vi "Configure Power Meter Settings.vi"(0 "VISA resource name":refnum<visa-resource-name>, 1 "Power Meter Average Count (10)":i32=10 min=2 max=1000, 2 "Power Meter Average State (0:Off)":i32(ring) items=["Off", "On"], 5 "Power Meter Frequency (1000000000Hz)":dbl=1000000000.0, 7 "Power Meter Offset State (0:Off)":i32(ring) items=["Off", "On"], 9 "Power Meter Offset (0.00dB)":dbl min=-100.0 max=100.0 step=0.01 format="%.2f", 11 "error in (no error)":errorcluster, 12 "Power Meter Range (0:Auto)":i32(ring) items=["Auto", "Low", "High"]) -> (4 "VISA resource name out":refnum<visa-resource-name>, 15 "error out":errorcluster)   [LabVIEW 2020, in "Anritsu Signal Analyzer Series.lvlib"]
doc: "Configures the Power Meter settings."
uses:
  Anritsu Signal Analyzer Series.lvlib
panel:
  # "Hz"
  # "dB"
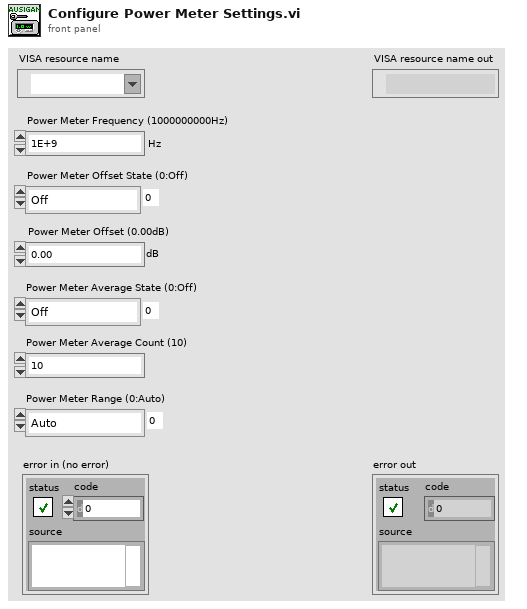
[diagram p1: front panel]
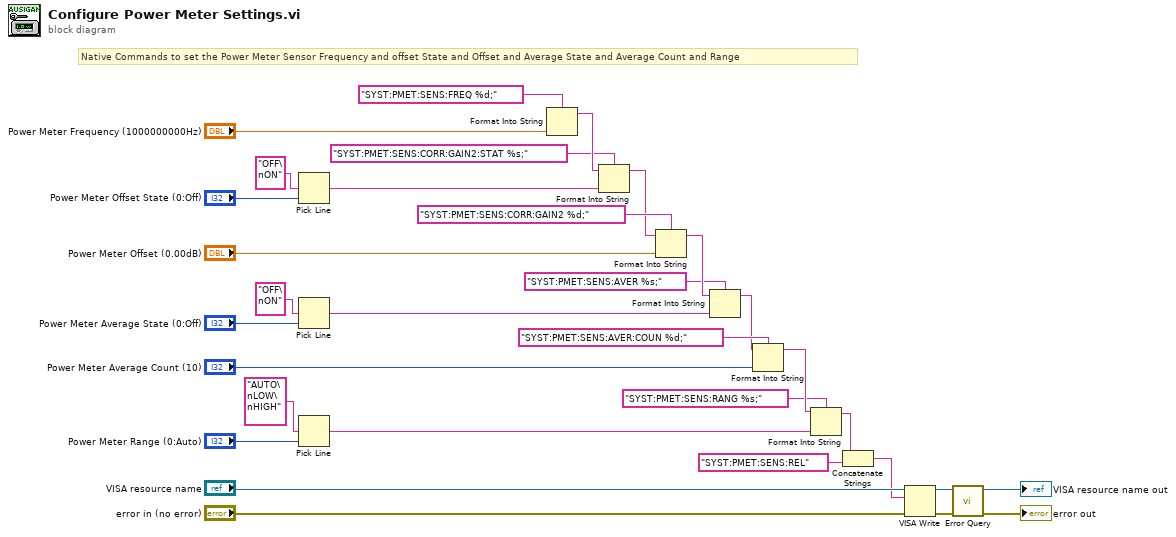
[diagram p0: block diagram]
diagram:
  # "Native Commands to set the Power Meter Sensor Frequency and offset State and Offset and Average State and Average Count and Range"
  n1 = Pick Line(multi-line string="OFF\nON" ("複数行文字列"), line index="Power Meter Offset State (0:Off)") -> (output string=w7:string)  [unwired: 1 in]
  n2 = Pick Line(multi-line string="OFF\nON" ("複数行文字列"), line index="Power Meter Average State (0:Off)") -> (output string=w5:string)  [unwired: 1 in]
  n3 = Pick Line(multi-line string="AUTO\nLOW\nHIGH" ("_Case0"), line index="Power Meter Range (0:Auto)") -> (output string=w3:string)  [unwired: 1 in]
  n4 = Format Into String(format string="SYST:PMET:SENS:FREQ %d;" ("形式文字列"), "Power Meter Frequency (1000000000Hz)") -> (resulting string=w22:string)  [unwired: 2 in, 1 out]
  n5 = Format Into String(format string="SYST:PMET:SENS:CORR:GAIN2:STAT %s;" ("_CommandSet"), initial string=w22, w7) -> (resulting string=w19:string)  [unwired: 1 in, 1 out]
  n6 = Format Into String(format string="SYST:PMET:SENS:CORR:GAIN2 %d;" ("形式文字列"), initial string=w19, "Power Meter Offset (0.00dB)") -> (resulting string=w18:string)  [unwired: 1 in, 1 out]
  n7 = Format Into String(format string="SYST:PMET:SENS:AVER %s;" ("_CommandSet"), initial string=w18, w5) -> (resulting string=w15:string)  [unwired: 1 in, 1 out]
  n8 = Format Into String(format string="SYST:PMET:SENS:AVER:COUN %d;" ("形式文字列"), initial string=w15, "Power Meter Average Count (10)") -> (resulting string=w14:string)  [unwired: 1 in, 1 out]
  n9 = Format Into String(format string="SYST:PMET:SENS:RANG %s;" ("_CommandSet"), initial string=w14, w3) -> (resulting string=w11:string)  [unwired: 1 in, 1 out]
  n10 = Concatenate Strings(w11, "SYST:PMET:SENS:REL") -> (w10:string)
  n11 = VISA Write(VISA resource name="VISA resource name", write buffer=w10, error in (no error)="error in (no error)") -> (VISA resource name out=w24:refnum<visa-resource-name>, error out=w23:errorcluster)  [unwired: 1 out]
  n12 = call "Error Query.vi"("error in (no error)"=w23, "VISA resource name"=w24) -> ("error out"=→"error out":errorcluster, "VISA resource name out"=→"VISA resource name out":refnum<visa-resource-name>)  [unwired: 6 in, 2 out]
